vi "InitGlobalLogQueue.vi"(8 "error in (no error)":errorcluster, 11 "TestCase in":refnum<class "testcase-CSMGlobalLog.lvclass">) -> (0 "error out":errorcluster, 2 "Global Log Queue":refnum<queue>, 3 "TestCase out":refnum<class "testcase-CSMGlobalLog.lvclass">)   [LabVIEW 2017, in "testcase-CSMGlobalLog.lvclass"]
uses:
  testcase-CSMGlobalLog.lvclass
  src/user.lib/_NEVSTOP/Communicable State Machine(CSM)/_Support/Typedef/_CSM_GlobalLog_MSG.ctl
  src/user.lib/_NEVSTOP/Communicable State Machine(CSM)/_Support/Typedef/_CSM_Response Source Message.ctl
  src/user.lib/_NEVSTOP/Communicable State Machine(CSM)/_Support/Typedef/_CSM_GlobalLog_MSG_TYPE.ctl
  testcase-CSMGlobalLog.lvclass/testcase-CSMGlobalLog.ctl
  GlobalVariable.vi
  src/user.lib/_NEVSTOP/Communicable State Machine(CSM)/Communicable State Machine.lvlib
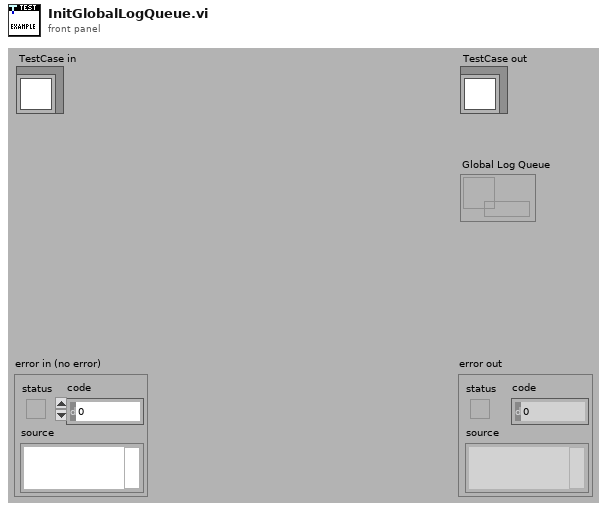
[diagram p1: front panel]
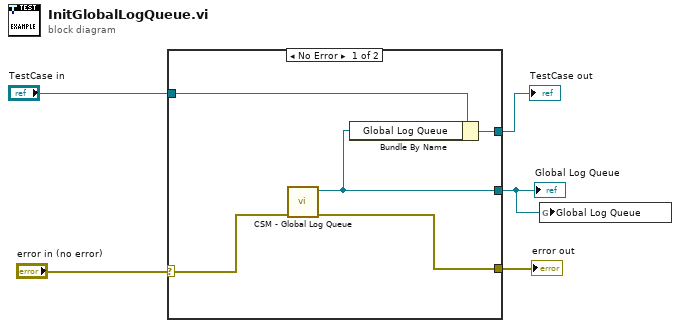
[diagram p0: block diagram]
diagram:
  n1 = case shown="No Error" "error in (no error)" {
    selector: "error in (no error)" -> [w9 w12]
    tunnel: [w7 _] -> w1
    tunnel: [w10 w12] -> w5
    tunnel: "TestCase in" -> [w8 w11]
    tunnel: [w6 w11] -> w2
    frame No Error {
      n2 = call "CSM - Global Log Queue.vi"("Error In"=w9) -> ("error out"=w10:errorcluster, "Global Log Queue"=w7:refnum<queue>)  [unwired: 9 in]
      n3 = Bundle By Name(cluster=w8, "Global Log Queue"=w7) -> (w6:refnum<class "testcase-CSMGlobalLog.lvclass">)
    }
    frame Error {
    }
  }
  "error out" <- w5
  "TestCase out" <- w2
  "Global Log Queue" <- w1
  n4 = global write "GlobalVariable.vi" "Global Log Queue"(w1) -> ()
